vi "algo.process.command.vi"(11 "algo.data.in":T1={"next.state"=enum."Wait.for.Command", "saved.state"=enum."Wait.for.Command", "scratch"={"i"=0, "n"=0, "start.addr"=0, "first.call?"=FALSE, "j"=0, "o"=0, "k"=0, "p"=0, "just.write"=FALSE, "orderId "=0, "dir"=0}, "mode"=enum."Get.Symbol", "cmd.mem.watchlist"={"read.request"=FALSE, "read.addr"=0, "read.ready"=FALSE, "val.watchlist.read"={"symbol"=0, "buy.start.addr"=0, "buy.size"=0, "buy.slots"=0, "sell.start.addr"=0, "sell.size"=0, "sell.slots"=0, "min.ask"=0, "max.bid"=0}, "write.request"=FALSE, "write.addr"=0, "val.watchlist.write"={"symbol"=0, "buy.start.addr"=0, "buy.size"=0, "buy.slots"=0, "sell.start.addr"=0, "sell.size"=0, "sell.slots"=0, "min.ask"=0, "max.bid"=0}}, "cmd.mem.orders"={"read.addr"=0, "read.request"=FALSE, "read.ready"=FALSE, "write.addr"=0, "write.request"=FALSE, "read.data"={"OrderId"=0, "Price"=0, "Quantity"=0}, "write.data"={"OrderId"=0, "Price"=0, "Quantity"=0}}, "cmd.state"={"write.to.state"=FALSE, "val.state"=[0, 0, 0, 0]}, "cmd.debug"={"write.to.debug"=FALSE, "val.debug"=[0, 0]}, "stats"={"min.ask"=0, "max.bid"=0, "price"=0, "quantity"=0, "execution"=FALSE}, "orderbook.command"={"type"=enum."AddOrder", "side"=0, "orderId "=0, "quantity"=0, "symbol"=0, "price"=0, "executed.qty"=0, "canceled.qty"=0, "remaining.qty"=0, "seconds"=0, "nanoseconds"=0, "Add"=FALSE, "Edit"=FALSE, "Remove"=FALSE}, "time"={"last"=0, "since"=0}, "watchlist.size"=0, "active.watchlist"={"item"={"symbol"=0, "buy.start.addr"=0, "buy.size"=0, "buy.slots"=0, "sell.start.addr"=0, "sell.size"=0, "sell.slots"=0, "min.ask"=0, "max.bid"=0}, "index"=0}, "active.order"={"buy"=FALSE, "sell"=FALSE, "addr"=0, "size"=0, "slots"=0, "index"=0}} {"active.watchlist"."item"."symbol" format="%.0x"; "cmd.mem.orders"."write.data"."OrderId" format="%.0x"; "cmd.mem.orders"."read.data"."OrderId" format="%.0x"; "cmd.mem.watchlist"."val.watchlist.write"."symbol" format="%.0x"; "cmd.mem.watchlist"."val.watchlist.read"."symbol" format="%.0x"}) -> (3 "algo.data.out":T1={"next.state"=enum."Wait.for.Command", "saved.state"=enum."Wait.for.Command", "scratch"={"i"=0, "n"=0, "start.addr"=0, "first.call?"=FALSE, "j"=0, "o"=0, "k"=0, "p"=0, "just.write"=FALSE, "orderId "=0, "dir"=0}, "mode"=enum."Get.Symbol", "cmd.mem.watchlist"={"read.request"=FALSE, "read.addr"=0, "read.ready"=FALSE, "val.watchlist.read"={"symbol"=0, "buy.start.addr"=0, "buy.size"=0, "buy.slots"=0, "sell.start.addr"=0, "sell.size"=0, "sell.slots"=0, "min.ask"=0, "max.bid"=0}, "write.request"=FALSE, "write.addr"=0, "val.watchlist.write"={"symbol"=0, "buy.start.addr"=0, "buy.size"=0, "buy.slots"=0, "sell.start.addr"=0, "sell.size"=0, "sell.slots"=0, "min.ask"=0, "max.bid"=0}}, "cmd.mem.orders"={"read.addr"=0, "read.request"=FALSE, "read.ready"=FALSE, "write.addr"=0, "write.request"=FALSE, "read.data"={"OrderId"=0, "Price"=0, "Quantity"=0}, "write.data"={"OrderId"=0, "Price"=0, "Quantity"=0}}, "cmd.state"={"write.to.state"=FALSE, "val.state"=[0, 0, 0, 0]}, "cmd.debug"={"write.to.debug"=FALSE, "val.debug"=[0, 0]}, "stats"={"min.ask"=0, "max.bid"=0, "price"=0, "quantity"=0, "execution"=FALSE}, "orderbook.command"={"type"=enum."AddOrder", "side"=0, "orderId "=0, "quantity"=0, "symbol"=0, "price"=0, "executed.qty"=0, "canceled.qty"=0, "remaining.qty"=0, "seconds"=0, "nanoseconds"=0, "Add"=FALSE, "Edit"=FALSE, "Remove"=FALSE}, "time"={"last"=0, "since"=0}, "watchlist.size"=0, "active.watchlist"={"item"={"symbol"=0, "buy.start.addr"=0, "buy.size"=0, "buy.slots"=0, "sell.start.addr"=0, "sell.size"=0, "sell.slots"=0, "min.ask"=0, "max.bid"=0}, "index"=0}, "active.order"={"buy"=FALSE, "sell"=FALSE, "addr"=0, "size"=0, "slots"=0, "index"=0}} {"active.watchlist"."item"."symbol" format="%.0x"; "cmd.mem.orders"."write.data"."OrderId" format="%.0x"; "cmd.mem.orders"."read.data"."OrderId" format="%.0x"; "cmd.mem.watchlist"."val.watchlist.write"."symbol" format="%.0x"; "cmd.mem.watchlist"."val.watchlist.read"."symbol" format="%.0x"})   [LabVIEW 2022 SP3]
uses:
  algo.data.ctl
  types/algo.states.ctl
  types/algo.scratch.ctl
  types/algo.mode.ctl
  types/algo.cmd.mem.watchlist.ctl
  types/algo.val.watchlist.ctl
  types/algo.cmd.mem.orders.ctl
  types/algo.val.order.ctl
  types/algo.cmd.state.ctl
  types/algo.val.state.ctl
  types/algo.cmd.debug.ctl
  types/algo.val.debug.ctl
  types/algo.stats.ctl
  common/orderbook.command.ctl
  common/orderbook.command.type.ctl
  types/algo.time.ctl
  <vilib>/rvi/DataTransferAndStorage/Container/Common/niFpgaContainerGetUniqueNameForEmu.vi
  <vilib>/rvi/DataTransferAndStorage/Container/Common/niFpgaContainerSetEmuInfo.vi
  <vilib>/rvi/eio/common/nirviEmuReportErrorAndStop.vi
  <vilib>/rvi/LocalResourceManager/LocalResourceManager.xnode
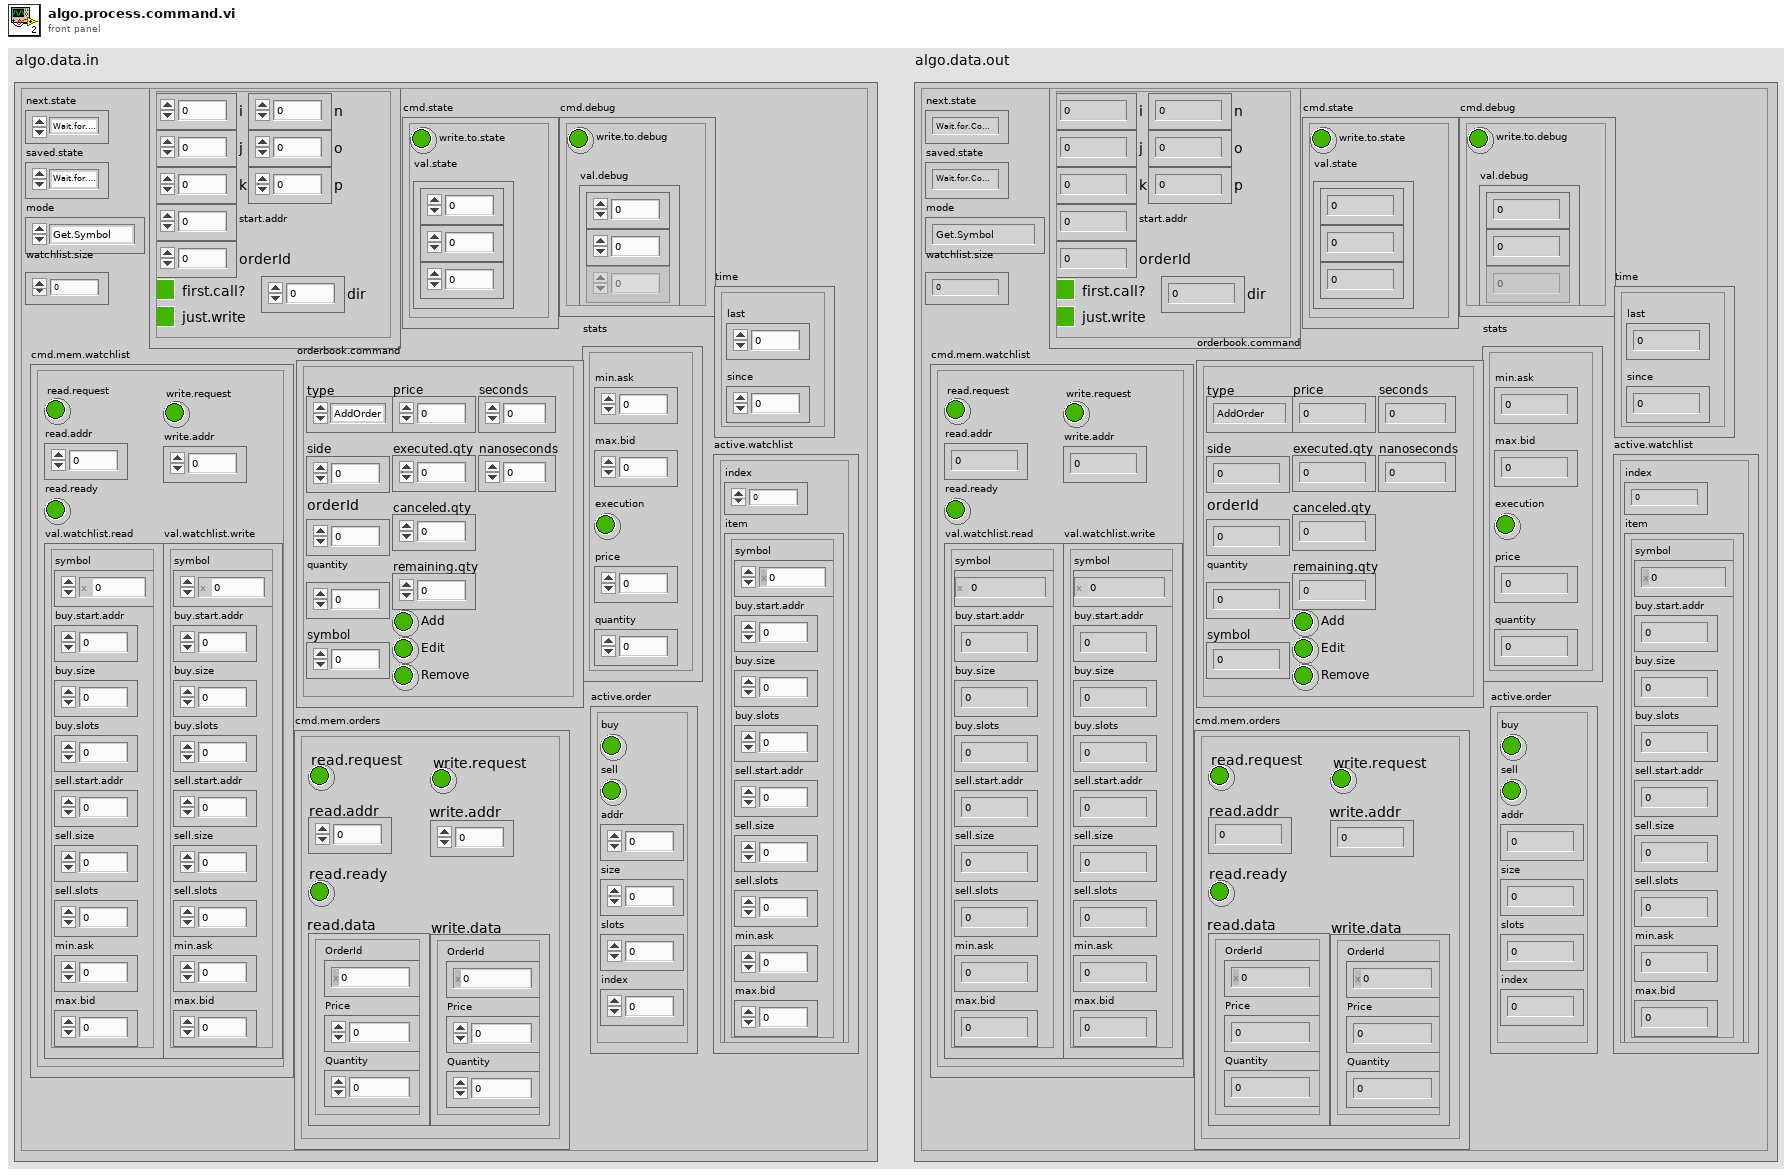
[diagram p1: front panel]
types:
  T1 = typedef "algo.data.ctl" = cluster{"next.state":T2, "saved.state":T2, "scratch":T3, "mode":T4, "cmd.mem.watchlist":T5, "cmd.mem.orders":T7, "cmd.state":T9, "cmd.debug":T11, "stats":T13, "orderbook.command":T14, "time":T16, "watchlist.size":u64, "active.watchlist":cluster{"item":T6, "index":u64}, "active.order":cluster{"buy":bool, "sell":bool, "addr":i16, "size":i16, "slots":i16, "index":i16}}
  T2 = typedef "algo.states.ctl" = enum16{"Noop", "Reset", "Configuration", "Debug", "Get.State", "Wait.for.Command", "Process.Command"}
  T3 = typedef "algo.scratch.ctl" = cluster{"i":u64, "n":u64, "start.addr":u16, "first.call?":bool, "j":u64, "o":u64, "k":u64, "p":u64, "just.write":bool, "orderId ":u64, "dir":i8}
  T4 = typedef "algo.mode.ctl" = enum16{"watchlist.iter", "order.buy.iter", "order.sell.iter", "Get.Symbol", "Search", "Shift"}
  T5 = typedef "algo.cmd.mem.watchlist.ctl" = cluster{"read.request":bool, "read.addr":u16, "read.ready":bool, "val.watchlist.read":T6, "write.request":bool, "write.addr":u16, "val.watchlist.write":T6}
  T6 = typedef "algo.val.watchlist.ctl" = cluster{"symbol":u64, "buy.start.addr":u16, "buy.size":u16, "buy.slots":u16, "sell.start.addr":u16, "sell.size":u16, "sell.slots":u16, "min.ask":u64, "max.bid":u64}
  T7 = typedef "algo.cmd.mem.orders.ctl" = cluster{"read.addr":u16, "read.request":bool, "read.ready":bool, "write.addr":u16, "write.request":bool, "read.data":T8, "write.data":T8}
  T8 = typedef "algo.val.order.ctl" = cluster{"OrderId":u64, "Price":u64, "Quantity":u32}
  T9 = typedef "algo.cmd.state.ctl" = cluster{"write.to.state":bool, "val.state":T10}
  T10 = typedef "algo.val.state.ctl" = u64[]
  T11 = typedef "algo.cmd.debug.ctl" = cluster{"write.to.debug":bool, "val.debug":T12}
  T12 = typedef "algo.val.debug.ctl" = u64[]
  T13 = typedef "algo.stats.ctl" = cluster{"min.ask":u32, "max.bid":u32, "price":u32, "quantity":u32, "execution":bool}
  T14 = typedef "orderbook.command.ctl" = cluster{"type":T15, "side":u8, "orderId ":u64, "quantity":u32, "symbol":u64, "price":u64, "executed.qty":u32, "canceled.qty":u32, "remaining.qty":u32, "seconds":u64, "nanoseconds":u64, "Add":bool, "Edit":bool, "Remove":bool}
  T15 = typedef "orderbook.command.type.ctl" = enum8{"Time", "AddOrder", "OrderExecuted", "OrderExecutedAtPrice", "ReduceSize", "ModifyOrder", "DeleteOrder", "Get.Everything", "Get.All.Orders", "Get.Top"}
  T16 = typedef "algo.time.ctl" = cluster{"last":u32, "since":u32}
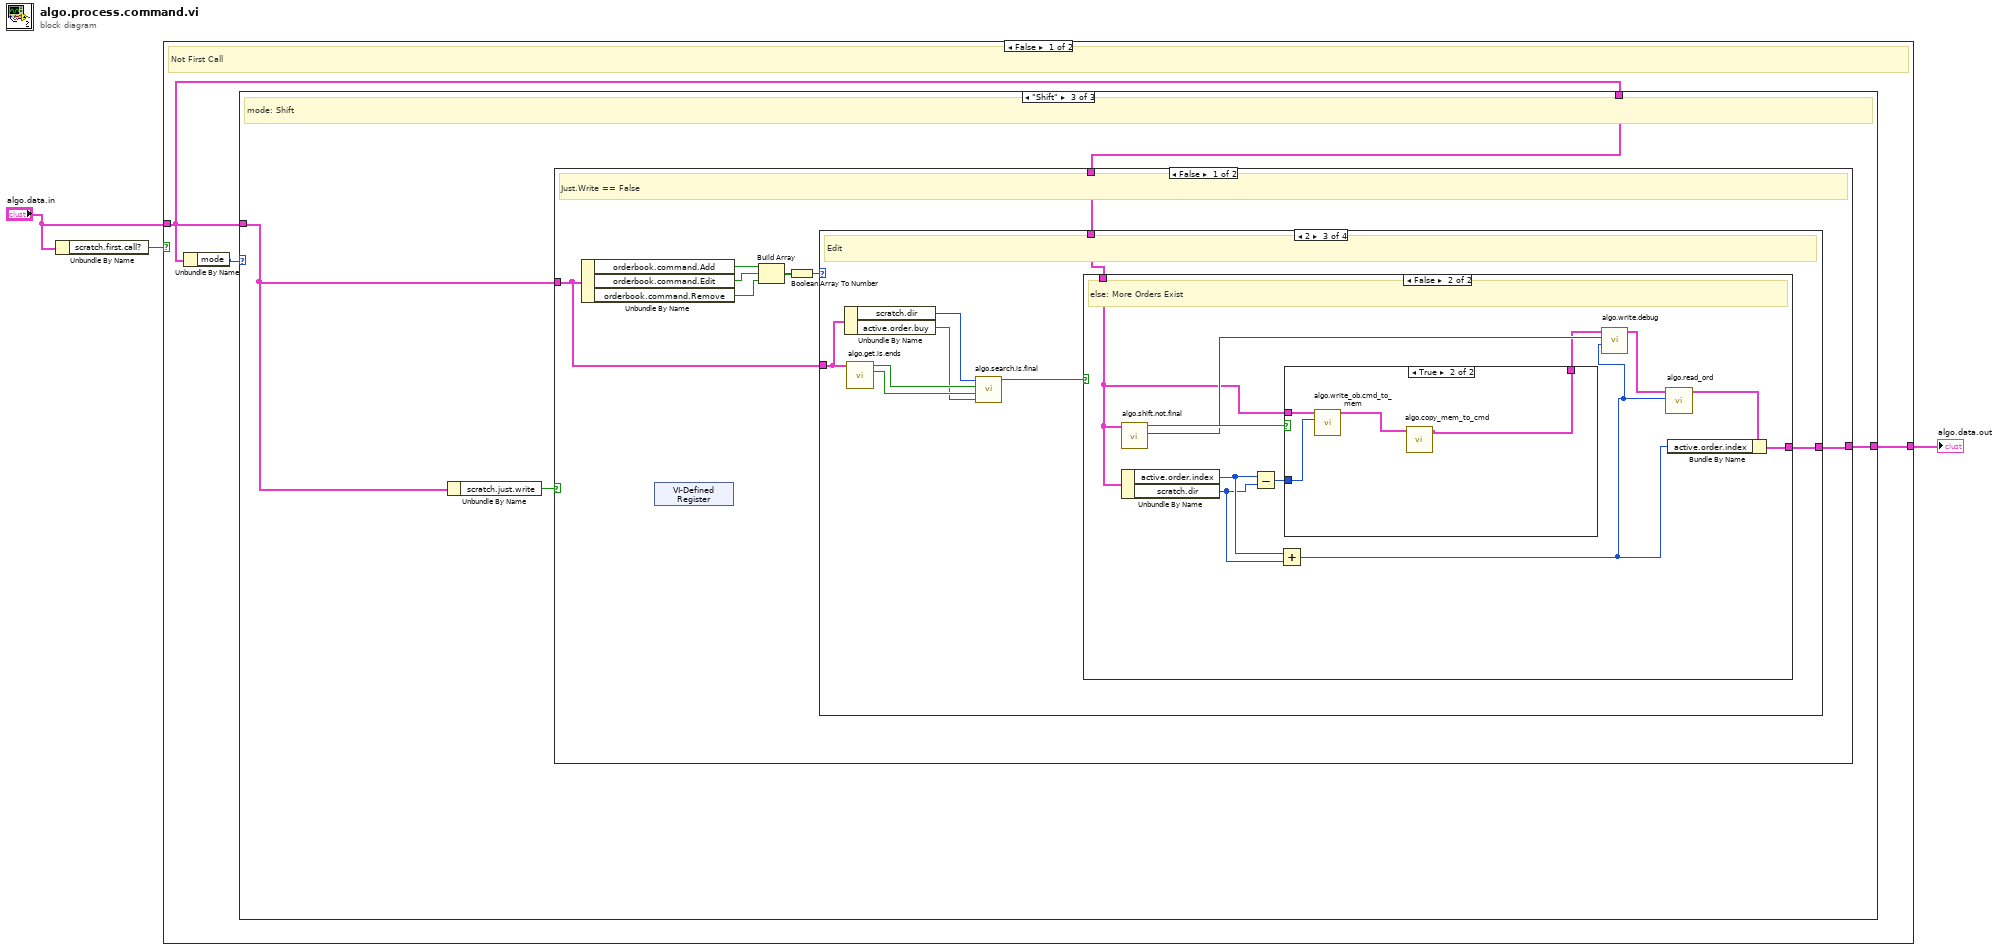
[diagram p0: block diagram]
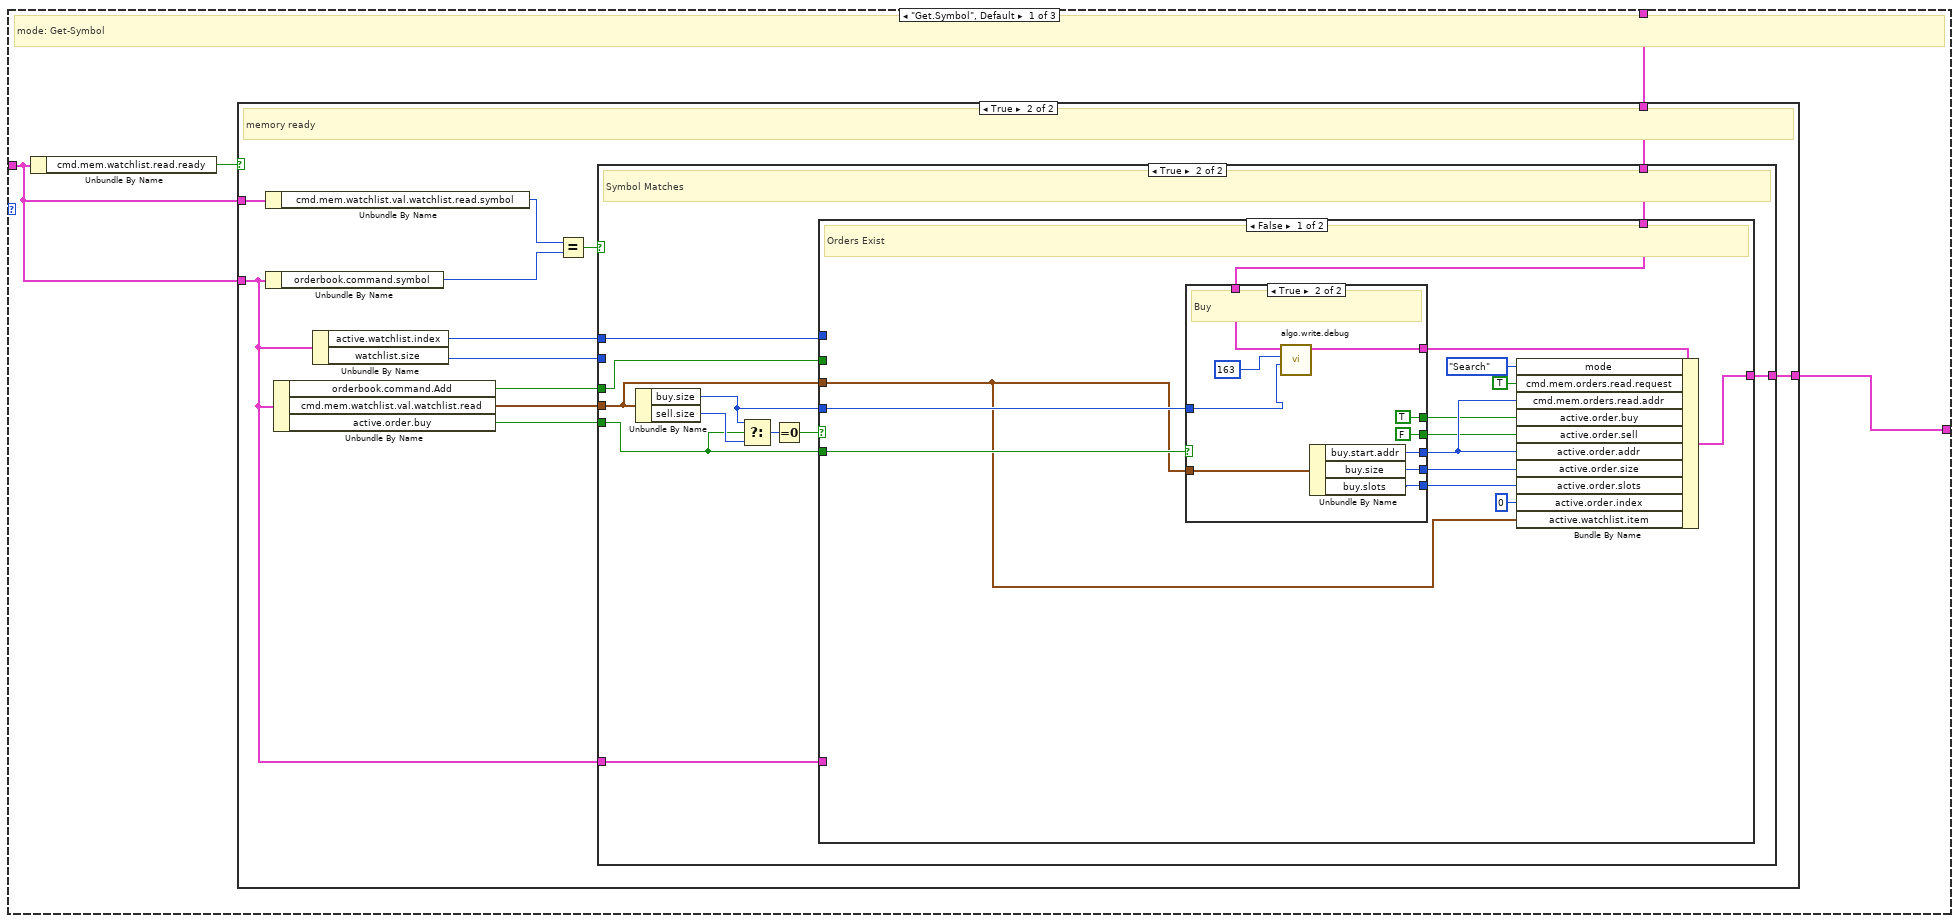
[diagram p2: hidden frame]
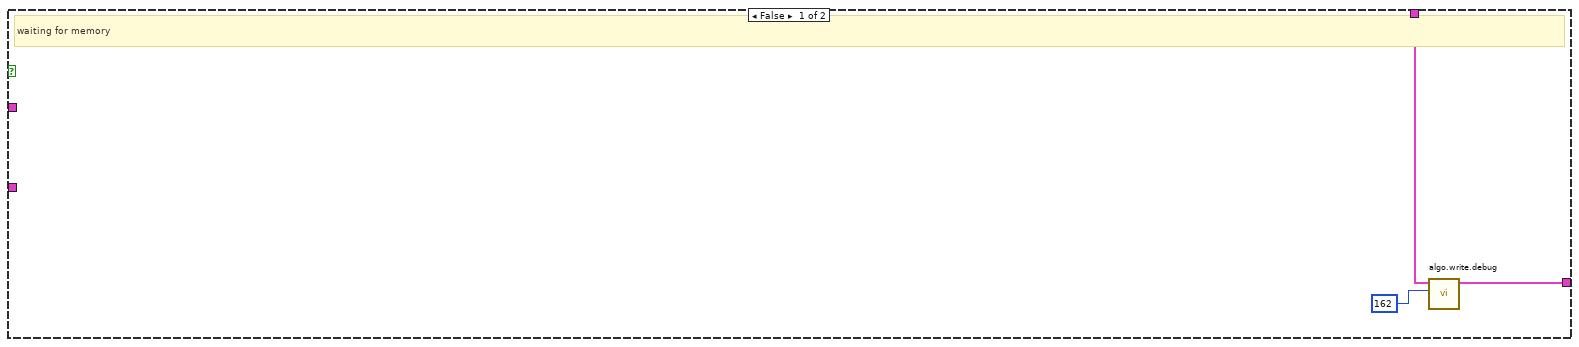
[diagram p3: hidden frame]
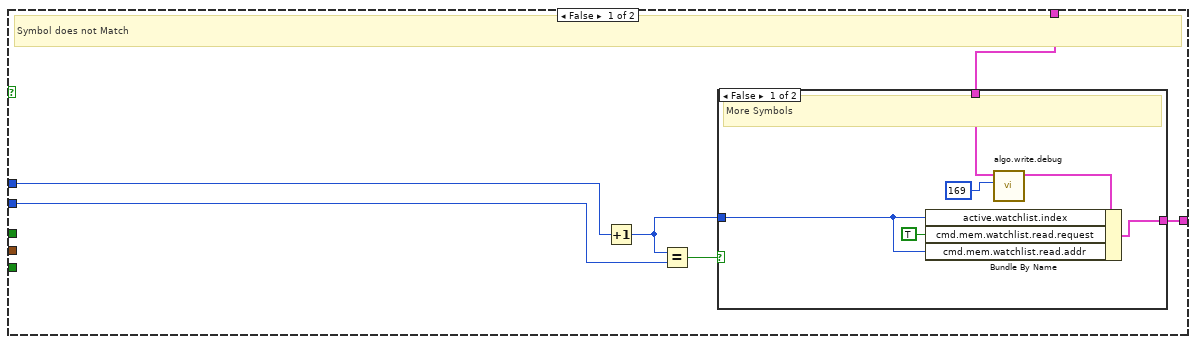
[diagram p4: hidden frame]
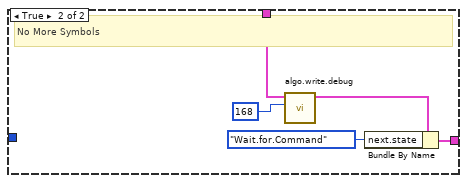
[diagram p5: hidden frame]
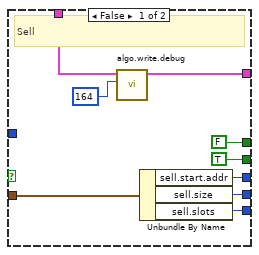
[diagram p6: hidden frame]
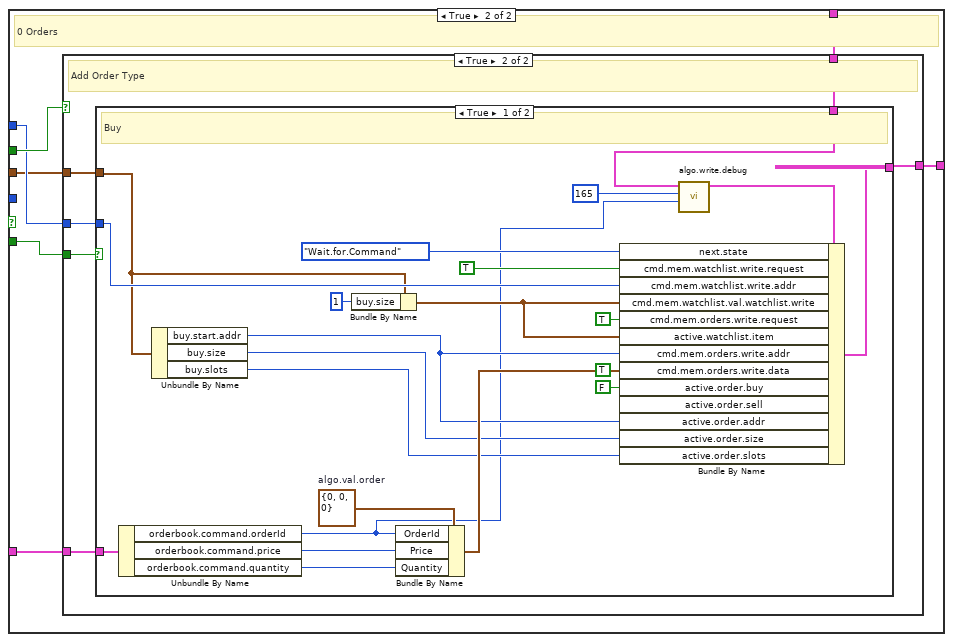
[diagram p7: hidden frame]
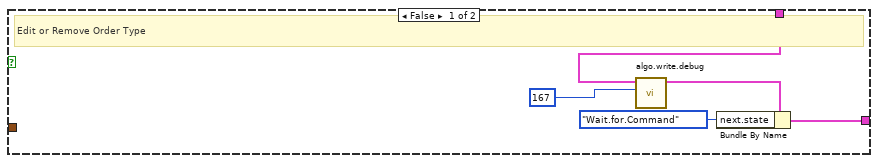
[diagram p8: hidden frame]
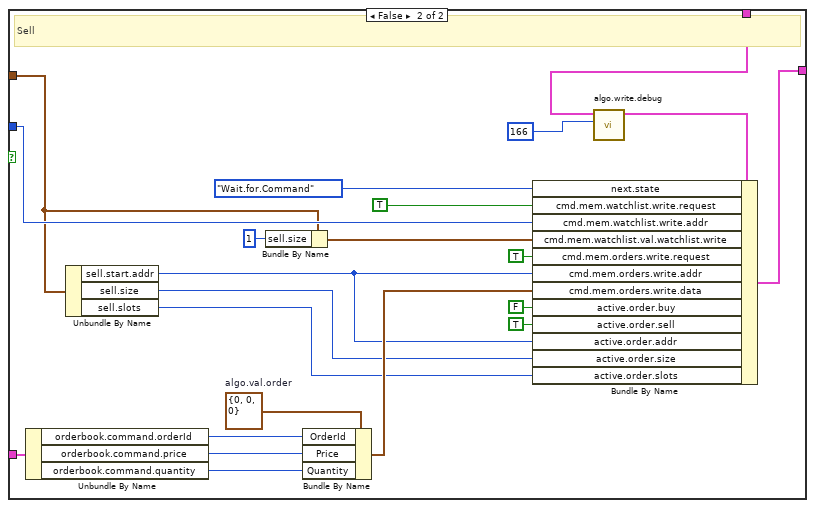
[diagram p9: hidden frame]
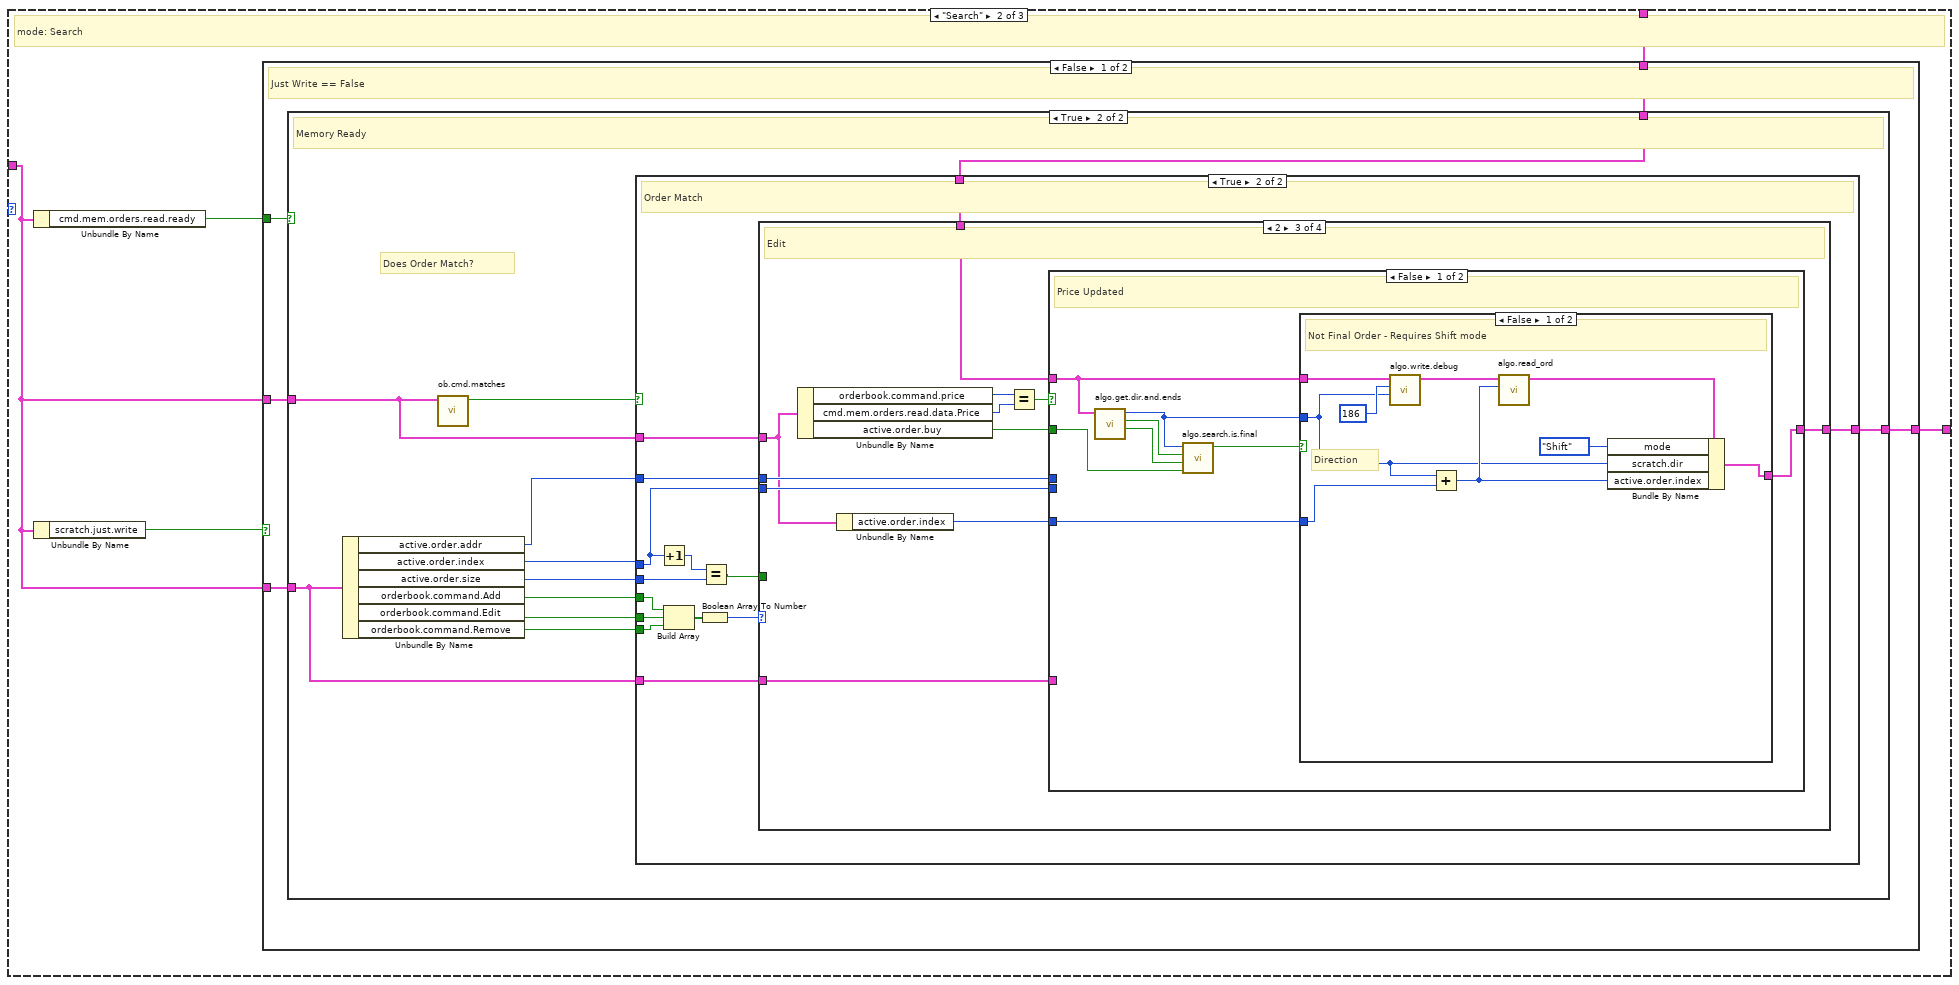
[diagram p10: hidden frame]
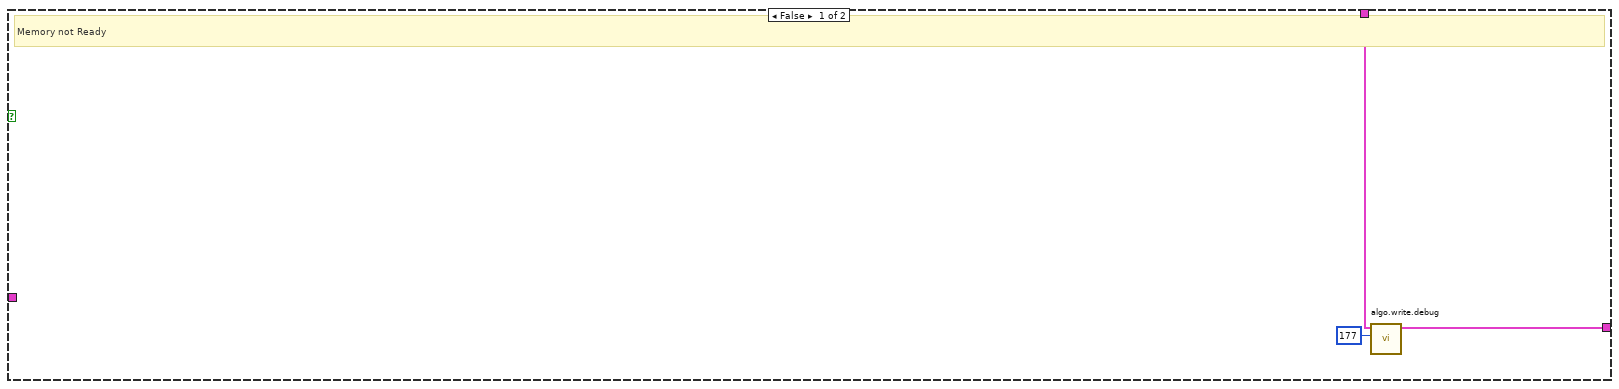
[diagram p11: hidden frame]
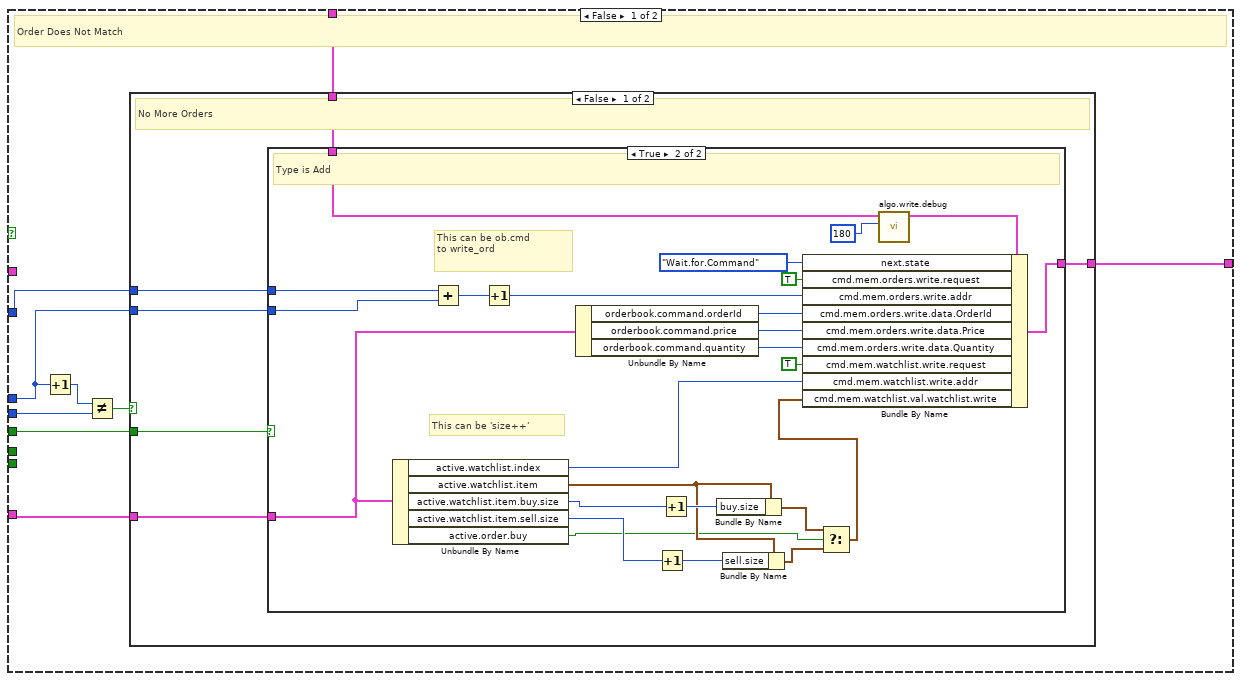
[diagram p12: hidden frame]
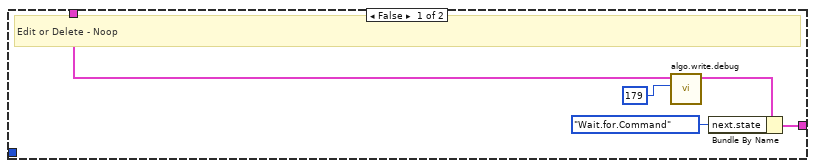
[diagram p13: hidden frame]
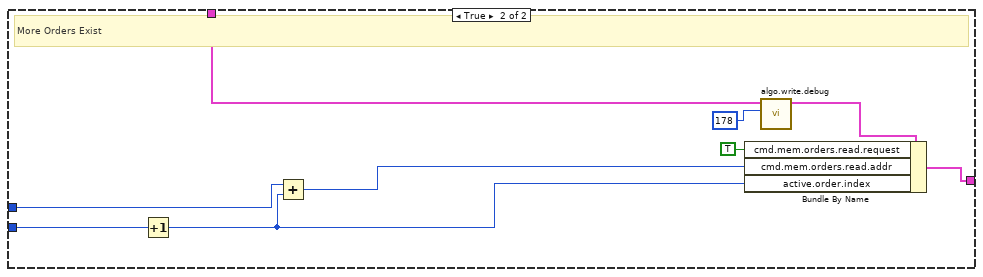
[diagram p14: hidden frame]
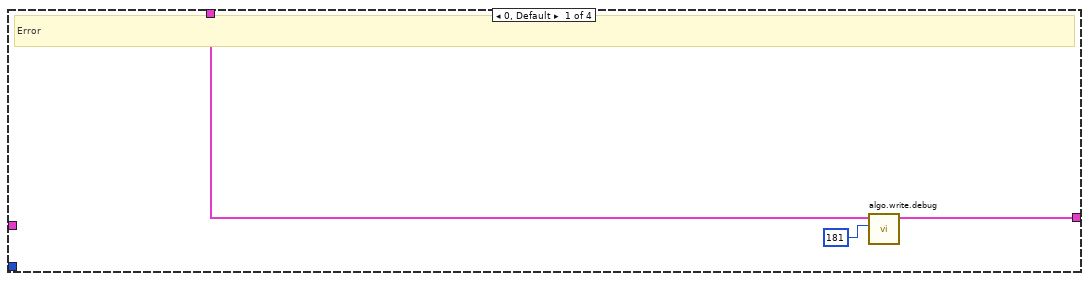
[diagram p15: hidden frame]
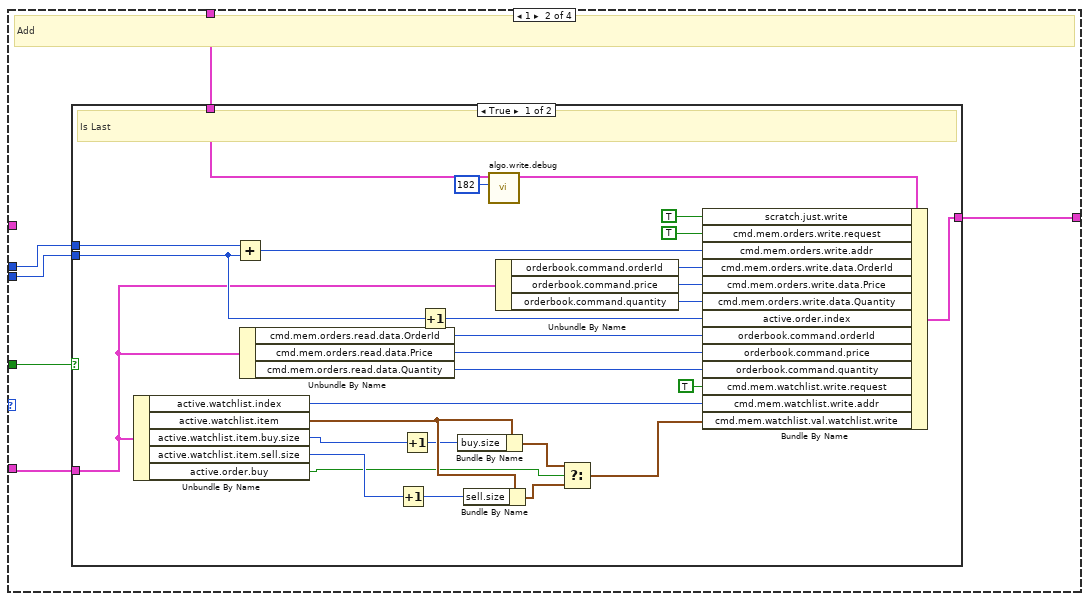
[diagram p16: hidden frame]
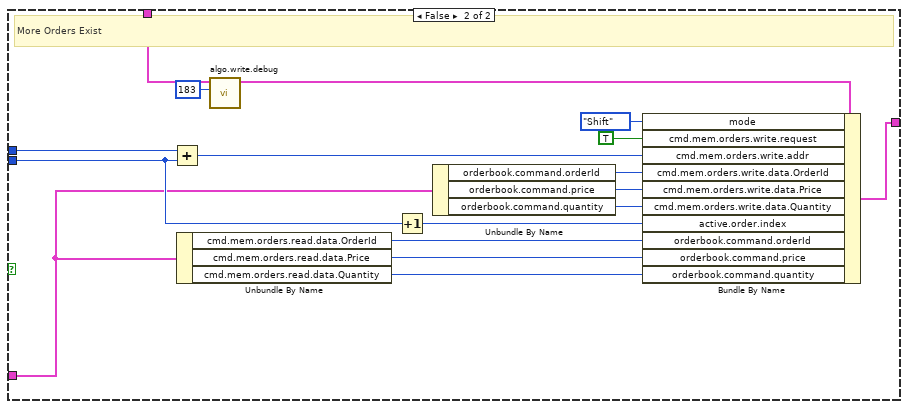
[diagram p17: hidden frame]
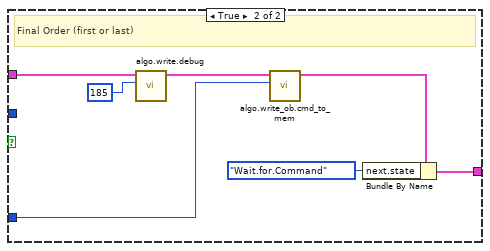
[diagram p18: hidden frame]
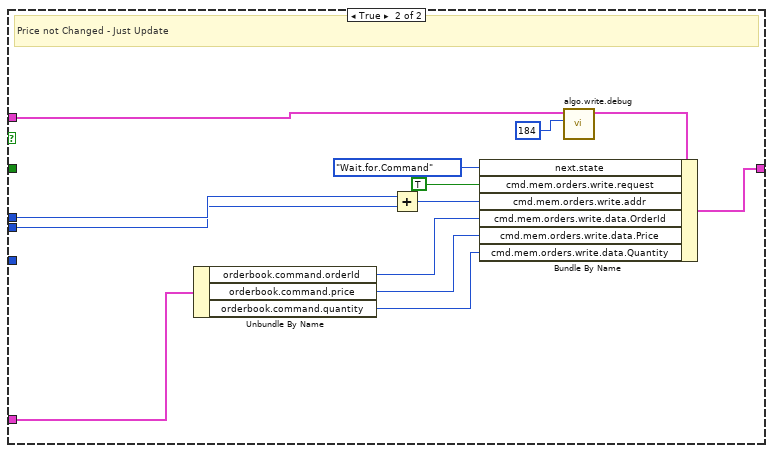
[diagram p19: hidden frame]
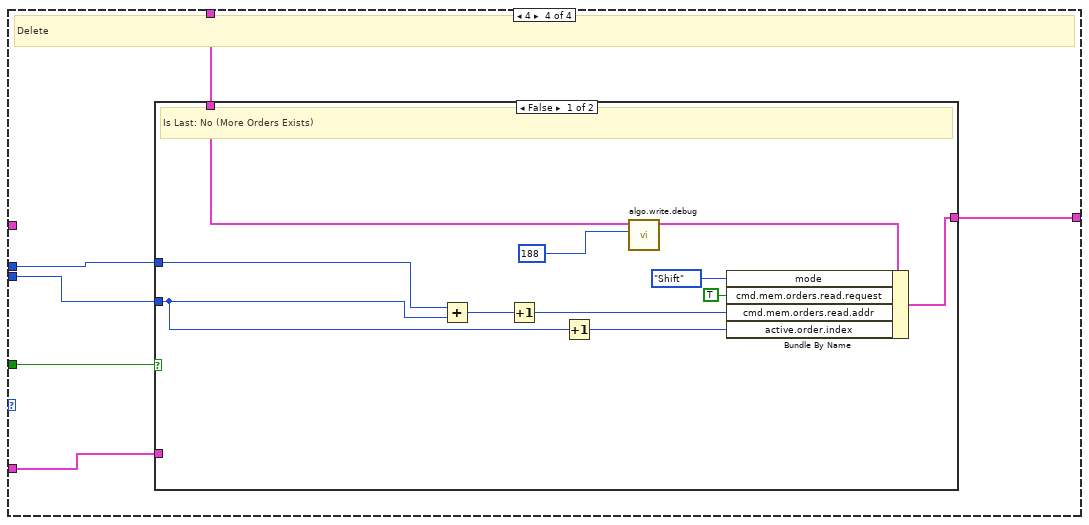
[diagram p20: hidden frame]
diagram:
  n1 = Unbundle By Name("algo.data.in") -> ("scratch.first.call?"=w3:bool)
  n2 = case shown="False" w3 {
    tunnel: [w4 w527] -> w2
    tunnel: "algo.data.in" -> [w5 w526]
    frame False {
      # "Not First Call"
      n3 = Unbundle By Name(w5) -> ("mode"=w6:T4)
      n4 = case shown="\"Shift\"" w6 {
        tunnel: w5 -> [w7 w149 w393]
        tunnel: w5 -> [w9 w153 w395]
        tunnel: [w8 w152 w394] -> w4
        frame "Get.Symbol", Default {
          # "mode: Get-Symbol"
          n5 = Unbundle By Name(w7) -> ("cmd.mem.watchlist.read.ready"=w10:bool)
          n6 = case shown="True" w10 {
            tunnel: w9 -> [w13 w19]
            tunnel: [w12 w18] -> w8
            tunnel: w7 -> [_ w25]
            tunnel: w7 -> [_ w14]
            frame False {
              # "waiting for memory"
              n7 = call "algo.write.debug.vi"("dbg.val.1"=u64 162, "algo.data.in"=w13) -> ("algo.data.out"=w12:T1)  [unwired: 9 in]
            }
            frame True {
              # "memory ready"
              n8 = Unbundle By Name(w25) -> ("cmd.mem.watchlist.val.watchlist.read.symbol"=w24:u64)
              n9 = Unbundle By Name(w14) -> ("orderbook.command.symbol"=w23:u64)
              n10 = Unbundle By Name(w14) -> ("orderbook.command.Add"=w15:bool, "cmd.mem.watchlist.val.watchlist.read"=w17:T6, "active.order.buy"=w16:bool)
              n11 = Unbundle By Name(w14) -> ("active.watchlist.index"=w20:u64, "watchlist.size"=w21:u64)
              n12 = Equal?(x=w24, y=w23) -> (x = y?=w22:bool)
              n13 = case shown="True" w22 {
                tunnel: w21 -> [w31 _]
                tunnel: w20 -> [w27 w47]
                tunnel: w19 -> [w29 w50]
                tunnel: [w28 w49] -> w18
                tunnel: w17 -> [_ w46]
                tunnel: w16 -> [_ w44]
                tunnel: w15 -> [_ w48]
                tunnel: w14 -> [_ w45]
                frame False {
                  # "Symbol does not Match"
                  n14 = Increment(x=w27) -> (x+1=w26:u64)
                  n15 = Equal?(x=w26, y=w31) -> (x = y?=w30:bool)
                  n16 = case shown="False" w30 {
                    tunnel: w29 -> [w34 w40]
                    tunnel: [w37 w42] -> w28
                    tunnel: w26 -> [w32 _]
                    frame False {
                      # "More Symbols"
                      n17 = call "algo.write.debug.vi"("dbg.val.1"=u64 169, "algo.data.in"=w34) -> ("algo.data.out"=w35:T1)  [unwired: 9 in]
                      n18 = Bundle By Name(cluster=w35, "active.watchlist.index"=w32, "cmd.mem.watchlist.read.request"=TRUE, "cmd.mem.watchlist.read.addr"=w32) -> (w37:T1)
                    }
                    frame True {
                      # "No More Symbols"
                      n19 = call "algo.write.debug.vi"("dbg.val.1"=u64 168, "algo.data.in"=w40) -> ("algo.data.out"=w39:T1)  [unwired: 9 in]
                      n20 = Bundle By Name(cluster=w39, "next.state"=algo.states."Wait.for.Command") -> (w42:T1)
                    }
                  }
                }
                frame True {
                  # "Symbol Matches"
                  n21 = Unbundle By Name(w46) -> ("buy.size"=w43:u16, "sell.size"=w53:u16)
                  n22 = Select(t=w43, s=w44, f=w53) -> (s? t:f=w52:u16)
                  n23 = Equal To 0?(x=w52) -> (x = 0?=w51:bool)
                  n24 = case shown="False" w51 {
                    tunnel: w48 -> [_ w93]
                    tunnel: w50 -> [w63 w92]
                    tunnel: [w67 w91] -> w49
                    tunnel: w47 -> [_ w90]
                    tunnel: w44 -> [w64 w89]
                    tunnel: w46 -> [w54 w88]
                    tunnel: w45 -> [_ w87]
                    tunnel: w43 -> [w55 _]
                    frame False {
                      # "Orders Exist"
                      n25 = case shown="True" w64 {
                        tunnel: w54 -> [w76 w86]
                        tunnel: [w75 w85] -> w61
                        tunnel: w63 -> [w73 w84]
                        tunnel: [w74 w83] -> w62
                        tunnel: [w71 w81] -> w60
                        tunnel: [w70 w80] -> w59
                        tunnel: [FALSE TRUE] -> w58
                        tunnel: [TRUE FALSE] -> w57
                        tunnel: w55 -> [_ w77]
                        frame False {
                          # "Sell"
                          n26 = call "algo.write.debug.vi"("dbg.val.1"=u64 164, "algo.data.in"=w73) -> ("algo.data.out"=w74:T1)  [unwired: 9 in]
                          n27 = Unbundle By Name(w76) -> ("sell.start.addr"=w75:u16, "sell.size"=w71:u16, "sell.slots"=w70:u16)
                        }
                        frame True {
                          # "Buy"
                          n28 = call "algo.write.debug.vi"("dbg.val.2"=w77, "dbg.val.1"=u64 163, "algo.data.in"=w84) -> ("algo.data.out"=w83:T1)  [unwired: 8 in]
                          n29 = Unbundle By Name(w86) -> ("buy.start.addr"=w85:u16, "buy.size"=w81:u16, "buy.slots"=w80:u16)
                        }
                      }
                      n30 = Bundle By Name(cluster=w62, "mode"=algo.mode."Search", "cmd.mem.orders.read.request"=TRUE, "cmd.mem.orders.read.addr"=w61, "active.order.buy"=w58, "active.order.sell"=w57, "active.order.addr"=w61, "active.order.size"=w60, "active.order.slots"=w59, "active.order.index"=i16 0, "active.watchlist.item"=w54) -> (w67:T1)
                    }
                    frame True {
                      # "0 Orders"
                      n31 = case shown="True" w93 {
                        tunnel: w92 -> [w95 w104]
                        tunnel: [w98 w103] -> w91
                        tunnel: w90 -> [_ w102]
                        tunnel: w89 -> [_ w101]
                        tunnel: w88 -> [_ w100]
                        tunnel: w87 -> [_ w99]
                        frame False {
                          # "Edit or Remove Order Type"
                          n32 = call "algo.write.debug.vi"("dbg.val.1"=u64 167, "algo.data.in"=w95) -> ("algo.data.out"=w96:T1)  [unwired: 9 in]
                          n33 = Bundle By Name(cluster=w96, "next.state"=algo.states."Wait.for.Command") -> (w98:T1)
                        }
                        frame True {
                          # "Add Order Type"
                          n34 = case shown="True" w101 {
                            tunnel: w104 -> [w110 w129]
                            tunnel: [w126 w148] -> w103
                            tunnel: w102 -> [w124 w146]
                            tunnel: w100 -> [w121 w142]
                            tunnel: w99 -> [w118 w139]
                            frame True {
                              w120 = T8 {"OrderId"=0, "Price"=0, "Quantity"=0}  # algo.val.order
                              # "Buy"
                              n35 = Unbundle By Name(w118) -> ("orderbook.command.orderId"=w105:u64, "orderbook.command.price"=w116:u64, "orderbook.command.quantity"=w117:u32)
                              n36 = Unbundle By Name(w121) -> ("buy.start.addr"=w113:u16, "buy.size"=w112:u16, "buy.slots"=w111:u16)
                              n37 = Bundle By Name(cluster=w121, "buy.size"=u16 1) -> (w106:T6)
                              n38 = Bundle By Name(cluster=w120, "OrderId"=w105, "Price"=w116, "Quantity"=w117) -> (w119:T8)
                              n39 = call "algo.write.debug.vi"("dbg.val.2"=w105, "dbg.val.1"=u64 165, "algo.data.in"=w110) -> ("algo.data.out"=w109:T1)  [unwired: 8 in]
                              n40 = Bundle By Name(cluster=w109, "next.state"=algo.states."Wait.for.Command", "cmd.mem.watchlist.write.request"=TRUE, "cmd.mem.watchlist.write.addr"=w124, "cmd.mem.watchlist.val.watchlist.write"=w106, "cmd.mem.orders.write.request"=TRUE, "active.watchlist.item"=w106, "cmd.mem.orders.write.addr"=w113, "cmd.mem.orders.write.data"=w119, "active.order.buy"=TRUE, "active.order.sell"=FALSE, "active.order.addr"=w113, "active.order.size"=w112, "active.order.slots"=w111) -> (w126:T1)
                            }
                            frame False {
                              w141 = T8 {"OrderId"=0, "Price"=0, "Quantity"=0}  # algo.val.order
                              # "Sell"
                              n41 = Unbundle By Name(w139) -> ("orderbook.command.orderId"=w136:u64, "orderbook.command.price"=w137:u64, "orderbook.command.quantity"=w138:u32)
                              n42 = Unbundle By Name(w142) -> ("sell.start.addr"=w135:u16, "sell.size"=w132:u16, "sell.slots"=w131:u16)
                              n43 = Bundle By Name(cluster=w142, "sell.size"=u16 1 ("buy.size")) -> (w144:T6)
                              n44 = Bundle By Name(cluster=w141, "OrderId"=w136, "Price"=w137, "Quantity"=w138) -> (w140:T8)
                              n45 = call "algo.write.debug.vi"("dbg.val.1"=u64 166, "algo.data.in"=w129) -> ("algo.data.out"=w130:T1)  [unwired: 9 in]
                              n46 = Bundle By Name(cluster=w130, "next.state"=algo.states."Wait.for.Command", "cmd.mem.watchlist.write.request"=TRUE, "cmd.mem.watchlist.write.addr"=w146, "cmd.mem.watchlist.val.watchlist.write"=w144, "cmd.mem.orders.write.request"=TRUE, "cmd.mem.orders.write.addr"=w135, "cmd.mem.orders.write.data"=w140, "active.order.buy"=FALSE, "active.order.sell"=TRUE, "active.order.addr"=w135, "active.order.size"=w132, "active.order.slots"=w131) -> (w148:T1)
                            }
                          }
                        }
                      }
                    }
                  }
                }
              }
            }
          }
        }
        frame "Search" {
          # "mode: Search"
          n47 = Unbundle By Name(w149) -> ("cmd.mem.orders.read.ready"=w151:bool)
          n48 = Unbundle By Name(w149) -> ("scratch.just.write"=w150:bool)
          n49 = case shown="False" w150 {
            tunnel: w153 -> [w158 w392]
            tunnel: [w157 w388] -> w152
            tunnel: w151 -> [w156 _]
            tunnel: w149 -> [w155 w386]
            tunnel: w149 -> [w154 _]
            frame False {
              # "Just Write == False"
              n50 = case shown="True" w156 {
                tunnel: w158 -> [w161 w166]
                tunnel: [w160 w167] -> w157
                tunnel: w155 -> [_ w164]
                tunnel: w154 -> [_ w162]
                frame False {
                  # "Memory not Ready"
                  n51 = call "algo.write.debug.vi"("dbg.val.1"=u64 177, "algo.data.in"=w161) -> ("algo.data.out"=w160:T1)  [unwired: 9 in]
                }
                frame True {
                  # "Does Order Match?"
                  # "Memory Ready"
                  n52 = Unbundle By Name(w164) -> ("active.order.addr"=w165:i16, "active.order.index"=w172:i16, "active.order.size"=w171:i16, "orderbook.command.Add"=w170:bool, "orderbook.command.Edit"=w169:bool, "orderbook.command.Remove"=w168:bool)
                  n53 = call "ob.cmd.matches.vi"("algo.data.in"=w162) -> ("OrderId.Matches"=w163:bool)  [unwired: 10 in]
                  n54 = case shown="True" w163 {
                    tunnel: w172 -> [w175 w230]
                    tunnel: w171 -> [w181 w234]
                    tunnel: w170 -> [w178 w238]
                    tunnel: w169 -> [_ w240]
                    tunnel: w168 -> [_ w237]
                    tunnel: [w176 w232] -> w167
                    tunnel: w166 -> [w177 w231]
                    tunnel: w165 -> [w174 w229]
                    tunnel: w164 -> [w173 w228]
                    tunnel: w162 -> [_ w227]
                    frame False {
                      # "Order Does Not Match"
                      n55 = Increment(x=w175) -> (x+1=w180:i16)
                      n56 = Not Equal?(x=w180, y=w181) -> (x != y?=w179:bool)
                      n57 = case shown="False" w179 {
                        tunnel: w178 -> [w187 _]
                        tunnel: w177 -> [w186 w223]
                        tunnel: [w185 w224] -> w176
                        tunnel: w175 -> [w184 w220]
                        tunnel: w174 -> [w183 w221]
                        tunnel: w173 -> [w182 _]
                        frame False {
                          # "No More Orders"
                          n58 = case shown="True" w187 {
                            tunnel: w186 -> [w191 w213]
                            tunnel: [w189 w215] -> w185
                            tunnel: w184 -> [_ w210]
                            tunnel: w183 -> [_ w211]
                            tunnel: w182 -> [_ w196]
                            frame False {
                              # "Edit or Delete - Noop"
                              n59 = call "algo.write.debug.vi"("dbg.val.1"=u64 179, "algo.data.in"=w191) -> ("algo.data.out"=w190:T1)  [unwired: 9 in]
                              n60 = Bundle By Name(cluster=w190, "next.state"=algo.states."Wait.for.Command") -> (w189:T1)
                            }
                            frame True {
                              # "This can be ob.cmd \nto write_ord"
                              # "This can be 'size++'"
                              # "Type is Add"
                              n61 = Unbundle By Name(w196) -> ("active.watchlist.index"=w194:u64, "active.watchlist.item"=w201:T6, "active.watchlist.item.buy.size"=w204:u16, "active.watchlist.item.sell.size"=w202:u16, "active.order.buy"=w197:bool)
                              n62 = Add(x=w211, y=w210) -> (x+y=w209:i16)
                              n63 = Increment(x=w209) -> (x+1=w208:i16)
                              n64 = Unbundle By Name(w196) -> ("orderbook.command.orderId"=w207:u64, "orderbook.command.price"=w206:u64, "orderbook.command.quantity"=w205:u32)
                              n65 = Increment(x=w202) -> (x+1=w200:u16)
                              n66 = Increment(x=w204) -> (x+1=w203:u16)
                              n67 = Bundle By Name(cluster=w201, "buy.size"=w203) -> (w199:T6)
                              n68 = Bundle By Name(cluster=w201, "sell.size"=w200) -> (w198:T6)
                              n69 = Select(t=w199, s=w197, f=w198) -> (s? t:f=w193:T6)
                              n70 = call "algo.write.debug.vi"("dbg.val.1"=u64 180, "algo.data.in"=w213) -> ("algo.data.out"=w214:T1)  [unwired: 9 in]
                              n71 = Bundle By Name(cluster=w214, "next.state"=algo.states."Wait.for.Command", "cmd.mem.orders.write.request"=TRUE, "cmd.mem.orders.write.addr"=w208, "cmd.mem.orders.write.data.OrderId"=w207, "cmd.mem.orders.write.data.Price"=w206, "cmd.mem.orders.write.data.Quantity"=w205, "cmd.mem.watchlist.write.request"=TRUE, "cmd.mem.watchlist.write.addr"=w194, "cmd.mem.watchlist.val.watchlist.write"=w193) -> (w215:T1)
                            }
                          }
                        }
                        frame True {
                          # "More Orders Exist"
                          n72 = Increment(x=w220) -> (x+1=w218:i16)
                          n73 = Add(x=w221, y=w218) -> (x+y=w219:i16)
                          n74 = call "algo.write.debug.vi"("dbg.val.1"=u64 178, "algo.data.in"=w223) -> ("algo.data.out"=w225:T1)  [unwired: 9 in]
                          n75 = Bundle By Name(cluster=w225, "cmd.mem.orders.read.request"=TRUE, "cmd.mem.orders.read.addr"=w219, "active.order.index"=w218) -> (w224:T1)
                        }
                      }
                    }
                    frame True {
                      # "Order Match"
                      n76 = Increment(x=w230) -> (x+1=w235:i16)
                      n77 = Build Array(w238, w240, w237) -> (w239:bool[])
                      n78 = Boolean Array To Number(Boolean array=w239) -> (number=w236:u8)
                      n79 = Equal?(x=w235, y=w234) -> (x = y?=w233:bool)
                      n80 = case shown="2" w236 {
                        tunnel: w233 -> [_ w249 _ w348]
                        tunnel: [w243 w247 w304 w347] -> w232
                        tunnel: w231 -> [w242 w248 w305 w346]
                        tunnel: w230 -> [_ w245 w302 w345]
                        tunnel: w229 -> [_ w246 w303 w344]
                        tunnel: w228 -> [_ w244 w301 w343]
                        tunnel: w227 -> [_ _ w296 _]
                        frame 0, Default {
                          # "Error"
                          n81 = call "algo.write.debug.vi"("dbg.val.1"=u64 181, "algo.data.in"=w242) -> ("algo.data.out"=w243:T1)  [unwired: 9 in]
                        }
                        frame 1 {
                          # "Add"
                          n82 = case shown="True" w249 {
                            tunnel: w248 -> [w277 w294]
                            tunnel: [w274 w291] -> w247
                            tunnel: w246 -> [w270 w287]
                            tunnel: w245 -> [w267 w284]
                            tunnel: w244 -> [w263 w279]
                            frame True {
                              # "Is Last"
                              n83 = Unbundle By Name(w263) -> ("active.watchlist.index"=w250:u64, "active.watchlist.item"=w259:T6, "active.watchlist.item.buy.size"=w261:u16, "active.watchlist.item.sell.size"=w260:u16, "active.order.buy"=w252:bool)
                              n84 = Add(x=w270, y=w267) -> (x+y=w269:i16)
                              n85 = Unbundle By Name(w263) -> ("cmd.mem.orders.read.data.OrderId"=w266:u64, "cmd.mem.orders.read.data.Price"=w265:u64, "cmd.mem.orders.read.data.Quantity"=w264:u32)
                              n86 = Increment(x=w260) -> (x+1=w258:u16)
                              n87 = Increment(x=w261) -> (x+1=w251:u16)
                              n88 = Increment(x=w267) -> (x+1=w253:i16)
                              n89 = Bundle By Name(cluster=w259, "buy.size"=w251) -> (w257:T6)
                              n90 = Bundle By Name(cluster=w259, "sell.size"=w258) -> (w256:T6)
                              n91 = call "algo.write.debug.vi"("dbg.val.1"=u64 182, "algo.data.in"=w277) -> ("algo.data.out"=w275:T1)  [unwired: 9 in]
                              n92 = Unbundle By Name(w263) -> ("orderbook.command.orderId"=w254:u64, "orderbook.command.price"=w272:u64, "orderbook.command.quantity"=w271:u32)
                              n93 = Select(t=w257, s=w252, f=w256) -> (s? t:f=w255:T6)
                              n94 = Bundle By Name(cluster=w275, "scratch.just.write"=TRUE, "cmd.mem.orders.write.request"=TRUE, "cmd.mem.orders.write.addr"=w269, "cmd.mem.orders.write.data.OrderId"=w254, "cmd.mem.orders.write.data.Price"=w272, "cmd.mem.orders.write.data.Quantity"=w271, "active.order.index"=w253, "orderbook.command.orderId"=w266, "orderbook.command.price"=w265, "orderbook.command.quantity"=w264, "cmd.mem.watchlist.write.request"=TRUE, "cmd.mem.watchlist.write.addr"=w250, "cmd.mem.watchlist.val.watchlist.write"=w255) -> (w274:T1)
                            }
                            frame False {
                              # "More Orders Exist"
                              n95 = Add(x=w287, y=w284) -> (x+y=w286:i16)
                              n96 = Unbundle By Name(w279) -> ("cmd.mem.orders.read.data.OrderId"=w282:u64, "cmd.mem.orders.read.data.Price"=w281:u64, "cmd.mem.orders.read.data.Quantity"=w280:u32)
                              n97 = call "algo.write.debug.vi"("dbg.val.1"=u64 183, "algo.data.in"=w294) -> ("algo.data.out"=w292:T1)  [unwired: 9 in]
                              n98 = Increment(x=w284) -> (x+1=w283:i16)
                              n99 = Unbundle By Name(w279) -> ("orderbook.command.orderId"=w290:u64, "orderbook.command.price"=w289:u64, "orderbook.command.quantity"=w288:u32)
                              n100 = Bundle By Name(cluster=w292, "mode"=algo.mode."Shift", "cmd.mem.orders.write.request"=TRUE, "cmd.mem.orders.write.addr"=w286, "cmd.mem.orders.write.data.OrderId"=w290, "cmd.mem.orders.write.data.Price"=w289, "cmd.mem.orders.write.data.Quantity"=w288, "active.order.index"=w283, "orderbook.command.orderId"=w282, "orderbook.command.price"=w281, "orderbook.command.quantity"=w280) -> (w291:T1)
                            }
                          }
                        }
                        frame 2 {
                          # "Edit"
                          n101 = Unbundle By Name(w296) -> ("orderbook.command.price"=w299:u64, "cmd.mem.orders.read.data.Price"=w300:u64, "active.order.buy"=w297:bool)
                          n102 = Unbundle By Name(w296) -> ("active.order.index"=w295:i16)
                          n103 = Equal?(x=w299, y=w300) -> (x = y?=w298:bool)
                          n104 = case shown="False" w298 {
                            tunnel: w305 -> [w312 w342]
                            tunnel: [w313 w339] -> w304
                            tunnel: w303 -> [_ w335]
                            tunnel: w302 -> [_ w334]
                            tunnel: w301 -> [_ w333]
                            tunnel: w297 -> [w309 _]
                            tunnel: w295 -> [w307 _]
                            frame False {
                              # "Price Updated"
                              n105 = call "algo.get.dir.and.ends.vi"("algo.data.in"=w312) -> ("isLast"=w310:bool, "isFirst"=w311:bool, "Direction"=w306:i8)  [unwired: 8 in]
                              n106 = call "algo.search.is.final.vi"("buy"=w309, "isLast"=w310, "isFirst"=w311, "Direction"=w306) -> ("isFinal"=w308:bool)  [unwired: 7 in]
                              n107 = case shown="False" w308 {
                                tunnel: w312 -> [w321 w328]
                                tunnel: [w320 w327] -> w313
                                tunnel: w307 -> [w318 w323]
                                tunnel: w306 -> [w314 _]
                                frame False {
                                # "Direction"
                                # "Not Final Order - Requires Shift mode"
                                n108 = call "algo.write.debug.vi"("dbg.val.2"=w314, "dbg.val.1"=u64 186, "algo.data.in"=w321) -> ("algo.data.out"=w317:T1)  [unwired: 8 in]
                                n109 = Add(x=w314, y=w318) -> (x+y=w315:i16)
                                n110 = call "algo.read_ord.vi"("index"=w315, "algo.data.in"=w317) -> ("algo.data.out"=w316:T1)  [unwired: 9 in]
                                n111 = Bundle By Name(cluster=w316, "mode"=algo.mode."Shift", "scratch.dir"=w314, "active.order.index"=w315) -> (w320:T1)
                                }
                                frame True {
                                # "Final Order (first or last)"
                                n112 = call "algo.write.debug.vi"("dbg.val.1"=u64 185, "algo.data.in"=w328) -> ("algo.data.out"=w325:T1)  [unwired: 9 in]
                                n113 = call "algo.write_ob.cmd_to_mem.vi"("index"=w323, "algo.data.in"=w325) -> ("algo.data.out"=w326:T1)  [unwired: 9 in]
                                n114 = Bundle By Name(cluster=w326, "next.state"=algo.states."Wait.for.Command") -> (w327:T1)
                                }
                              }
                            }
                            frame True {
                              # "Price not Changed - Just Update"
                              n115 = Unbundle By Name(w333) -> ("orderbook.command.orderId"=w332:u64, "orderbook.command.price"=w331:u64, "orderbook.command.quantity"=w330:u32)
                              n116 = Add(x=w335, y=w334) -> (x+y=w336:i16)
                              n117 = call "algo.write.debug.vi"("dbg.val.1"=u64 184, "algo.data.in"=w342) -> ("algo.data.out"=w340:T1)  [unwired: 9 in]
                              n118 = Bundle By Name(cluster=w340, "next.state"=algo.states."Wait.for.Command", "cmd.mem.orders.write.request"=TRUE, "cmd.mem.orders.write.addr"=w336, "cmd.mem.orders.write.data.OrderId"=w332, "cmd.mem.orders.write.data.Price"=w331, "cmd.mem.orders.write.data.Quantity"=w330) -> (w339:T1)
                            }
                          }
                        }
                        frame 4 {
                          # "Delete"
                          n119 = case shown="False" w348 {
                            tunnel: [w358 w372] -> w347
                            tunnel: w346 -> [w356 w371]
                            tunnel: w345 -> [w353 _]
                            tunnel: w344 -> [w352 _]
                            tunnel: w343 -> [_ w368]
                            frame False {
                              # "Is Last: No (More Orders Exists)"
                              n120 = Add(x=w352, y=w353) -> (x+y=w351:i16)
                              n121 = Increment(x=w351) -> (x+1=w350:i16)
                              n122 = Increment(x=w353) -> (x+1=w349:i16)
                              n123 = call "algo.write.debug.vi"("dbg.val.1"=u64 188, "algo.data.in"=w356) -> ("algo.data.out"=w357:T1)  [unwired: 9 in]
                              n124 = Bundle By Name(cluster=w357, "mode"=algo.mode."Shift", "cmd.mem.orders.read.request"=TRUE, "cmd.mem.orders.read.addr"=w350, "active.order.index"=w349) -> (w358:T1)
                            }
                            frame True {
                              # "Is Last"
                              n125 = Unbundle By Name(w368) -> ("active.order.buy"=w364:bool, "active.order.size"=w363:i16, "active.watchlist.index"=w365:u64)
                              n126 = call "algo.write.debug.vi"("dbg.val.1"=u64 187, "algo.data.in"=w371) -> ("algo.data.out"=w361:T1)  [unwired: 9 in]
                              n127 = Unbundle By Name(w361) -> ("active.watchlist.item"=w360:T6)
                              n128 = Decrement(x=w363) -> (x-1=w362:i16)
                              n129 = case shown="True" w364 {
                                tunnel: [w375 w378] -> w366
                                tunnel: w362 -> [w374 w377]
                                tunnel: w360 -> [w373 w376]
                                frame False {
                                n130 = Bundle By Name(cluster=w373, "sell.size"=w374) -> (w375:T6)
                                }
                                frame True {
                                n131 = Bundle By Name(cluster=w376, "buy.size"=w377) -> (w378:T6)
                                }
                              }
                              n132 = Bundle By Name(cluster=w361, "next.state"=algo.states."Wait.for.Command", "cmd.mem.watchlist.write.request"=TRUE, "cmd.mem.watchlist.val.watchlist.write"=w366, "cmd.mem.watchlist.write.addr"=w365) -> (w372:T1)
                            }
                          }
                        }
                      }
                    }
                  }
                }
              }
            }
            frame True {
              # "Just Write"
              n133 = Unbundle By Name(w386) -> ("active.order.addr"=w384:i16, "active.order.index"=w383:i16, "orderbook.command.orderId"=w379:u64, "orderbook.command.price"=w382:u64, "orderbook.command.quantity"=w381:u32)
              n134 = Add(x=w384, y=w383) -> (x+y=w385:i16)
              n135 = call "algo.write.debug.vi"("dbg.val.2"=w379, "dbg.val.1"=u64 176, "algo.data.in"=w392) -> ("algo.data.out"=w390:T1)  [unwired: 8 in]
              n136 = Bundle By Name(cluster=w390, "next.state"=algo.states."Wait.for.Command", "scratch.just.write"=FALSE, "cmd.mem.orders.write.request"=TRUE, "cmd.mem.orders.write.addr"=w385, "cmd.mem.orders.write.data.OrderId"=w379, "cmd.mem.orders.write.data.Price"=w382, "cmd.mem.orders.write.data.Quantity"=w381) -> (w388:T1)
            }
          }
        }
        frame "Shift" {
          # "mode: Shift"
          n137 = Unbundle By Name(w393) -> ("scratch.just.write"=w396:bool)
          n138 = case shown="False" w396 {
            tunnel: w395 -> [w397 w523]
            tunnel: [w398 w525] -> w394
            tunnel: w393 -> [w399 w516]
            frame False {
              # "Just.Write == False"
              n139 = Unbundle By Name(w399) -> ("orderbook.command.Add"=w403:bool, "orderbook.command.Edit"=w402:bool, "orderbook.command.Remove"=w401:bool)
              n140 = xnode "VI-Defined Register"() -> ()  [unwired: 1 out]
              n141 = Build Array(w403, w402, w401) -> (w404:bool[])
              n142 = Boolean Array To Number(Boolean array=w404) -> (number=w400:u8)
              n143 = case shown="2" w400 {
                tunnel: w399 -> [_ w413 w444 w490]
                tunnel: [w405 w415 w448 w489] -> w398
                tunnel: w397 -> [w407 w414 w449 w487]
                frame 0, Default {
                  # "Error"
                  n144 = call "algo.write.debug.vi"("dbg.val.1"=u64 203, "algo.data.in"=w407) -> ("algo.data.out"=w408:T1)  [unwired: 9 in]
                  n145 = Bundle By Name(cluster=w408, "next.state"=algo.states."Wait.for.Command") -> (w405:T1)
                }
                frame 1 {
                  # "Add"
                  n146 = Unbundle By Name(w413) -> ("active.order.index"=w410:i16, "active.order.size"=w417:i16, "active.order.addr"=w411:i16)
                  n147 = Increment(x=w410) -> (x+1=w412:i16)
                  n148 = Equal?(x=w412, y=w417) -> (x = y?=w416:bool)
                  n149 = case shown="True" w416 {
                    tunnel: [w423 w440] -> w415
                    tunnel: w414 -> [w424 w439]
                    tunnel: w413 -> [_ w432]
                    tunnel: w410 -> [w422 w433]
                    tunnel: w411 -> [w418 _]
                    frame False {
                      # "Is Last == Fale"
                      n150 = call "algo.write.debug.vi"("dbg.val.1"=u64 204, "algo.data.in"=w424) -> ("algo.data.out"=w426:T1)  [unwired: 9 in]
                      n151 = Add(x=w422, y=w418) -> (x+y=w420:i16)
                      n152 = call "algo.write_ob.cmd_to_mem.vi"("index"=w422, "algo.data.in"=w426) -> ("algo.data.out"=w425:T1)  [unwired: 9 in]
                      n153 = Increment(x=w422) -> (x+1=w427:i16)
                      n154 = Increment(x=w420) -> (x+1=w419:i16)
                      n155 = Bundle By Name(cluster=w425, "active.order.index"=w427, "cmd.mem.orders.read.request"=TRUE, "cmd.mem.orders.read.addr"=w419) -> (w423:T1)
                    }
                    frame True {
                      # "Is Last == True"
                      n156 = call "algo.write.debug.vi"("dbg.val.1"=u64 205, "algo.data.in"=w439) -> ("algo.data.out"=w436:T1)  [unwired: 9 in]
                      n157 = Unbundle By Name(w432) -> ("cmd.mem.orders.read.data.OrderId"=w429:u64, "cmd.mem.orders.read.data.Price"=w430:u64, "cmd.mem.orders.read.data.Quantity"=w431:u32)
                      n158 = call "algo.inc_sym_size_and_write_sym.vi"("algo.data.in"=w436) -> ("algo.data.out"=w435:T1)  [unwired: 10 in]
                      n159 = Increment(x=w433) -> (x+1=w437:i16)
                      n160 = call "algo.write_ob.cmd_to_mem.vi"("index"=w433, "algo.data.in"=w435) -> ("algo.data.out"=w434:T1)  [unwired: 9 in]
                      n161 = Bundle By Name(cluster=w434, "scratch.just.write"=TRUE, "active.order.index"=w437, "orderbook.command.orderId"=w429, "orderbook.command.price"=w430, "orderbook.command.quantity"=w431) -> (w440:T1)
                    }
                  }
                }
                frame 2 {
                  # "Edit"
                  n162 = Unbundle By Name(w444) -> ("scratch.dir"=w442:i8, "active.order.buy"=w443:bool)
                  n163 = call "algo.get.is.ends.vi"("algo.data.in"=w444) -> ("isLast"=w447:bool, "isFirst"=w446:bool)  [unwired: 9 in]
                  n164 = call "algo.search.is.final.vi"("buy"=w443, "isLast"=w447, "isFirst"=w446, "Direction"=w442) -> ("isFinal"=w445:bool)  [unwired: 7 in]
                  n165 = case shown="False" w445 {
                    tunnel: w449 -> [w455 w475]
                    tunnel: [w460 w478] -> w448
                    frame True {
                      # "Is Final Order in List"
                      n166 = call "algo.shift.final.vi"("algo.data.in"=w455) -> ("dbg.val.1"=w456:u64, "write_ob.cmd"=w457:bool)  [unwired: 9 in]
                      n167 = Unbundle By Name(w455) -> ("active.order.index"=w452:i16, "scratch.dir"=w451:i8)
                      n168 = Subtract(x=w452, y=w451) -> (x-y=w454:i16)
                      n169 = Add(x=w452, y=w451) -> (x+y=w450:i16)
                      n170 = case shown="False" w457 {
                        tunnel: w455 -> [w463 w467]
                        tunnel: w454 -> [w462 w466]
                        tunnel: [w461 w464] -> w453
                        frame False {
                          n171 = call "algo.write_mem.ord_to_mem.vi"("index"=w462, "algo.data.in"=w463) -> ("algo.data.out"=w461:T1)  [unwired: 9 in]
                        }
                        frame True {
                          n172 = call "algo.write_ob.cmd_to_mem.vi"("index"=w466, "algo.data.in"=w467) -> ("algo.data.out"=w465:T1)  [unwired: 9 in]
                          n173 = call "algo.copy_mem_to_cmd.vi"("algo.data.in"=w465) -> ("algo.data.out"=w464:T1)  [unwired: 10 in]
                        }
                      }
                      n174 = call "algo.write.debug.vi"("dbg.val.1"=w456, "algo.data.in"=w453) -> ("algo.data.out"=w459:T1)  [unwired: 9 in]
                      n175 = Bundle By Name(cluster=w459, "scratch.just.write"=TRUE, "active.order.index"=w450) -> (w460:T1)
                    }
                    frame False {
                      # "else: More Orders Exist"
                      n176 = call "algo.shift.not.final.vi"("algo.data.in"=w475) -> ("dbg.val.1"=w476:u64, "write_ob.cmd"=w477:bool)  [unwired: 9 in]
                      n177 = Unbundle By Name(w475) -> ("active.order.index"=w472:i16, "scratch.dir"=w471:i8)
                      n178 = Subtract(x=w472, y=w471) -> (x-y=w474:i16)
                      n179 = Add(x=w472, y=w471) -> (x+y=w468:i16)
                      n180 = case shown="True" w477 {
                        tunnel: w475 -> [w481 w485]
                        tunnel: w474 -> [w480 w484]
                        tunnel: [w479 w482] -> w473
                        frame False {
                          n181 = call "algo.write_mem.ord_to_mem.vi"("index"=w480, "algo.data.in"=w481) -> ("algo.data.out"=w479:T1)  [unwired: 9 in]
                        }
                        frame True {
                          n182 = call "algo.write_ob.cmd_to_mem.vi"("index"=w484, "algo.data.in"=w485) -> ("algo.data.out"=w483:T1)  [unwired: 9 in]
                          n183 = call "algo.copy_mem_to_cmd.vi"("algo.data.in"=w483) -> ("algo.data.out"=w482:T1)  [unwired: 10 in]
                        }
                      }
                      n184 = call "algo.write.debug.vi"("dbg.val.2"=w468, "dbg.val.1"=w476, "algo.data.in"=w473) -> ("algo.data.out"=w470:T1)  [unwired: 8 in]
                      n185 = call "algo.read_ord.vi"("index"=w468, "algo.data.in"=w470) -> ("algo.data.out"=w469:T1)  [unwired: 9 in]
                      n186 = Bundle By Name(cluster=w469, "active.order.index"=w468) -> (w478:T1)
                    }
                  }
                }
                frame 4 {
                  # "Delete"
                  n187 = Unbundle By Name(w490) -> ("active.order.index"=w486:i16, "active.order.size"=w492:i16)
                  n188 = Increment(x=w486) -> (x+1=w491:i16)
                  n189 = Equal?(x=w491, y=w492) -> (x = y?=w488:bool)
                  n190 = case shown="True" w488 {
                    tunnel: [w494 w508] -> w489
                    tunnel: w487 -> [w498 w506]
                    tunnel: w486 -> [w497 w507]
                    frame False {
                      # "Is Last == Fale"
                      n191 = call "algo.write.debug.vi"("dbg.val.1"=u64 194, "algo.data.in"=w498) -> ("algo.data.out"=w500:T1)  [unwired: 9 in]
                      n192 = Decrement(x=w497) -> (x-1=w499:i16)
                      n193 = call "algo.write_ob.cmd_to_mem.vi"("index"=w499, "algo.data.in"=w500) -> ("algo.data.out"=w496:T1)  [unwired: 9 in]
                      n194 = Increment(x=w497) -> (x+1=w493:i16)
                      n195 = call "algo.read_ord.vi"("index"=w493, "algo.data.in"=w496) -> ("algo.data.out"=w495:T1)  [unwired: 9 in]
                      n196 = Bundle By Name(cluster=w495, "active.order.index"=w493) -> (w494:T1)
                    }
                    frame True {
                      # "Is Last == True"
                      n197 = call "algo.write.debug.vi"("dbg.val.1"=u64 193, "algo.data.in"=w506) -> ("algo.data.out"=w505:T1)  [unwired: 9 in]
                      n198 = call "algo.dec_sym_size_and_write_sym.vi"("algo.data.in"=w505) -> ("algo.data.out"=w504:T1)  [unwired: 10 in]
                      n199 = Decrement(x=w507) -> (x-1=w502:i16)
                      n200 = call "algo.write_ob.cmd_to_mem.vi"("index"=w502, "algo.data.in"=w504) -> ("algo.data.out"=w509:T1)  [unwired: 9 in]
                      n201 = Bundle By Name(cluster=w509, "next.state"=algo.states."Wait.for.Command") -> (w508:T1)
                    }
                  }
                }
              }
            }
            frame True {
              w515 = T8 {"OrderId"=0, "Price"=0, "Quantity"=0}  # algo.val.order
              # "write_ob.cmd_to_mem()"
              # "Just.Write == True"
              n202 = Unbundle By Name(w516) -> ("active.order.addr"=w520:i16, "active.order.index"=w519:i16)
              n203 = Unbundle By Name(w516) -> ("orderbook.command.orderId"=w513:u64, "orderbook.command.price"=w512:u64, "orderbook.command.quantity"=w511:u32)
              n204 = Add(x=w520, y=w519) -> (x+y=w517:i16)
              n205 = Bundle By Name(cluster=w515, "OrderId"=w513, "Price"=w512, "Quantity"=w511) -> (w514:T8)
              n206 = call "algo.write.debug.vi"("dbg.val.1"=u64 192, "algo.data.in"=w523) -> ("algo.data.out"=w522:T1)  [unwired: 9 in]
              n207 = Bundle By Name(cluster=w522, "next.state"=algo.states."Wait.for.Command", "cmd.mem.orders.write.request"=TRUE, "cmd.mem.orders.write.addr"=w517, "cmd.mem.orders.write.data"=w514) -> (w525:T1)
            }
          }
        }
      }
    }
    frame True {
      # "First Call"
      n208 = Unbundle By Name(w526) -> ("watchlist.size"=w529:u64)
      n209 = Equal To 0?(x=w529) -> (x = 0?=w528:bool)
      n210 = case shown="False" w528 {
        tunnel: w526 -> [w539 w546]
        tunnel: [w543 w548] -> w527
        tunnel: w526 -> [w536 _]
        frame False {
          w532 = u8 131  # const.S
          w534 = u8 102  # const.B
          w530 = u64 0 ("scratch.i")
          # "Change mode\nRequest 1st symbol"
          # "Symbols in Watchlist"
          n211 = Unbundle By Name(w536) -> ("orderbook.command.side"=w531:u8)
          n212 = Equal?(x=w534, y=w531) -> (x = y?=w535:bool)
          n213 = Equal?(x=w531, y=w532) -> (x = y?=w533:bool)
          n214 = call "algo.write.debug.vi"("dbg.val.1"=u64 161, "algo.data.in"=w539) -> ("algo.data.out"=w538:T1)  [unwired: 9 in]
          n215 = Bundle By Name(cluster=w538, "scratch.first.call?"=FALSE, "mode"=algo.mode."Get.Symbol", "active.watchlist.index"=w530, "cmd.mem.watchlist.read.request"=TRUE, "cmd.mem.watchlist.read.addr"=w530, "active.order.buy"=w535, "active.order.sell"=w533) -> (w543:T1)
        }
        frame True {
          # "Exit -> Go back to Wait.for.Command state"
          # "No Symbols in Watchlist"
          n216 = call "algo.write.debug.vi"("dbg.val.1"=u64 160, "algo.data.in"=w546) -> ("algo.data.out"=w545:T1)  [unwired: 9 in]
          n217 = Bundle By Name(cluster=w545, "next.state"=algo.states."Wait.for.Command") -> (w548:T1)
        }
      }
    }
  }
  "algo.data.out" <- w2
